vi "composeChipKick.vi"(4 "Game in":refnum<class "Game.lvclass">, 6 "Distance to target":dbl, 8 "error in (no error)":errorcluster, 9 "kick_z":dbl, 10 "kick_x":dbl, 11 "KickToSkill in":refnum<class "KickToSkill.lvclass">) -> (0 "error out":errorcluster, 1 "kick_z out":dbl, 2 "kick_x out":dbl, 3 "KickToSkill out":refnum<class "KickToSkill.lvclass">)   [LabVIEW 2021, in "KickToSkill.lvclass"]
uses:
  KickToSkill.lvclass
  Game_class/Game.lvclass
  Game_class/Game.lvclass/Game.ctl
  Team_class/OffensivePlay.ctl
  Team_class/Team.lvclass/Team.ctl
  Object_class/Object.lvclass/Object.ctl
  <vilib>/Analysis/baseanly.llb/Unit Vector (DBL).vi
  Object_class/Read x.vi
  Team_class/Read OffensivePlay.vi
  Game_class/Read BallRef.vi
  Game_class/Read FieldRef.vi
  Game_class/Read NewParameters.vi
  Game_class/Read OffensiveTeam.vi
  Ball_class/Ball.lvclass
  D:/RoboIme/horie/SSL_AI/Object_class/Object.lvclass
  Ally_class/Ally.lvclass
  D:/RoboIme/horie/SSL_AI/Team_class/Team.lvclass
  Field_class/Field.lvclass
  <vilib>/Analysis/NI_AALBase.lvlib
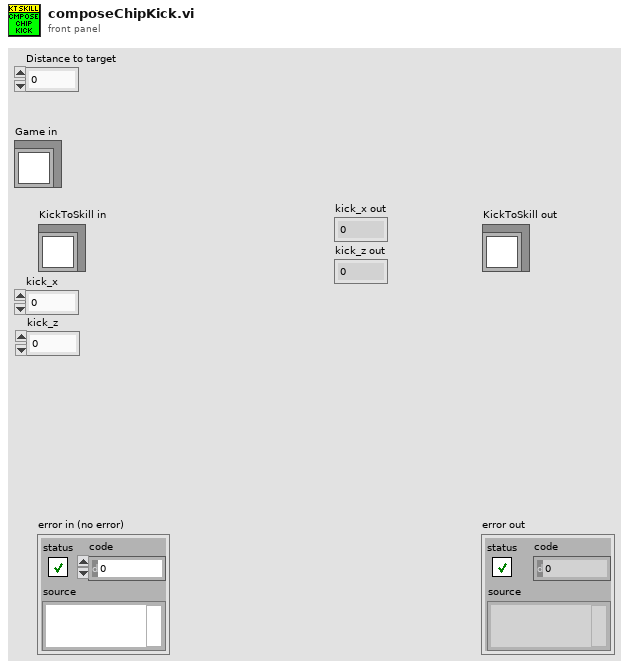
[diagram p1: front panel]
types:
  T1 = typedef "NewParameters.ctl" = cluster{"PenaltyDistance":dbl, "DistanceAttackerToBackBall":dbl, "Division":enum16{"Div B", "Div A"}, "DistanceToAvoidyEnemyRobot":dbl, "BallPlacementDistance":dbl, "DisatanceBehindBallToStealBall":dbl, "MaxDistanceToPositionKickoff":dbl, "BlockEnemyTarget":bool, "MaxStopVAng":dbl, "DistanceMarkerToEnemy":dbl, "IgnoreDribblerContact":bool, "DistanceToBeginEnemyPosession":dbl, "GoToBallWhenEnemyNotMoving":bool, "EnemyDistanceToReduceVelocity":dbl, "TurnOnEnemyDistanceToReduceVelocity":bool, "EnemyDistanceToShootOutBall":dbl, "DefenseKickBall":bool, "MoreKickToGoal? (0-0.3)":dbl, "ChipKickInEnemyField":bool, "ShootOutRobotId":dbl, "FieldLenghtDenominatorInShootOut":dbl, "AdjustPositionInBallPlacement":bool, "PowerGodPass":dbl, "VelocityAbortEnemyPos":dbl, "MaxDistToBeginPass":dbl, "MinDistToBeginPass":dbl, "VelocityInDirects":dbl, "BadDribblerIDs":i32[], "NewKickToDistanceAroundBall":dbl, "PowerAvoidColisionMarker":dbl, "DistanceToAvoidColisionMarker":dbl, "AvoidBallKick":dbl, "DistanceTryKick":dbl, "SuicideKickDIstance":dbl, "FirstKickAtck":bool, "AdjustFirstKickDistance":dbl, "FirstKickDefense":bool, "AvoidAimLessKick":dbl, "DistanceToAvoidyEnemyShootRobot ":dbl, "NumberOfMarkers":dbl, "PotField":bool, "PIDLateral":bool, "MinDistanceFirstKickX":dbl, "MinDistanceFirstKickY":dbl, "FractionOfDistToTouchGround\nAfterChipKick":dbl, "FractionOfKickxWhen\nComposedWithKickz":dbl, "Style":T2, "MoveInTurnState":bool, "DistFromEnemyToConsider\nMoveInTurnState":dbl, "CascadePID":bool, "TurnAroundParameters":cluster{"Radius":dbl, "Multiplier":dbl, "ChordAngle":dbl}, "SafeDriveVel":dbl, "DistanceToGoToBackBall":dbl}
  T2 = typedef "Style.ctl" = enum16{"Insanity", "Offensive", "Defensive"}
  T3 = typedef "OffensivePlay.ctl" = enum16{"5RobotsPassGamePlay", "5PreparePassGame", "5RobotsKeeperGame", "KeeperPassToStriker", "5RobotsNormalGamePlay", "PrepareKeeperPass", "ACBPass", "ABCPass", "PrepareTriplePass", "TableWithStriker", "TableWith2ndStrikerPlay", "PrepareDoublePass", "PrepareRollToPass", "SimplePass", "PreparePass", "PassToStriker", "BallOutOfField", "PassTo2ndStriker", "StopOffensive", "Prepare Penalty Enemy", "EnemyPossessionAtEnemyField", "EnemyPossesionAtOurField", "TestPlay", "PreparePenaltyAlly", "KickPenaltyAlly", "PrepareKickoffAlly", "PrepareKickoffEnemy", "IndirectEnemy", "DirectEnemy", "PreparePassInGame1", "NormalGame", "DirectKick", "Pass", "Halt", "Timeout", "PassPlay", "PenaltyEnemy"}
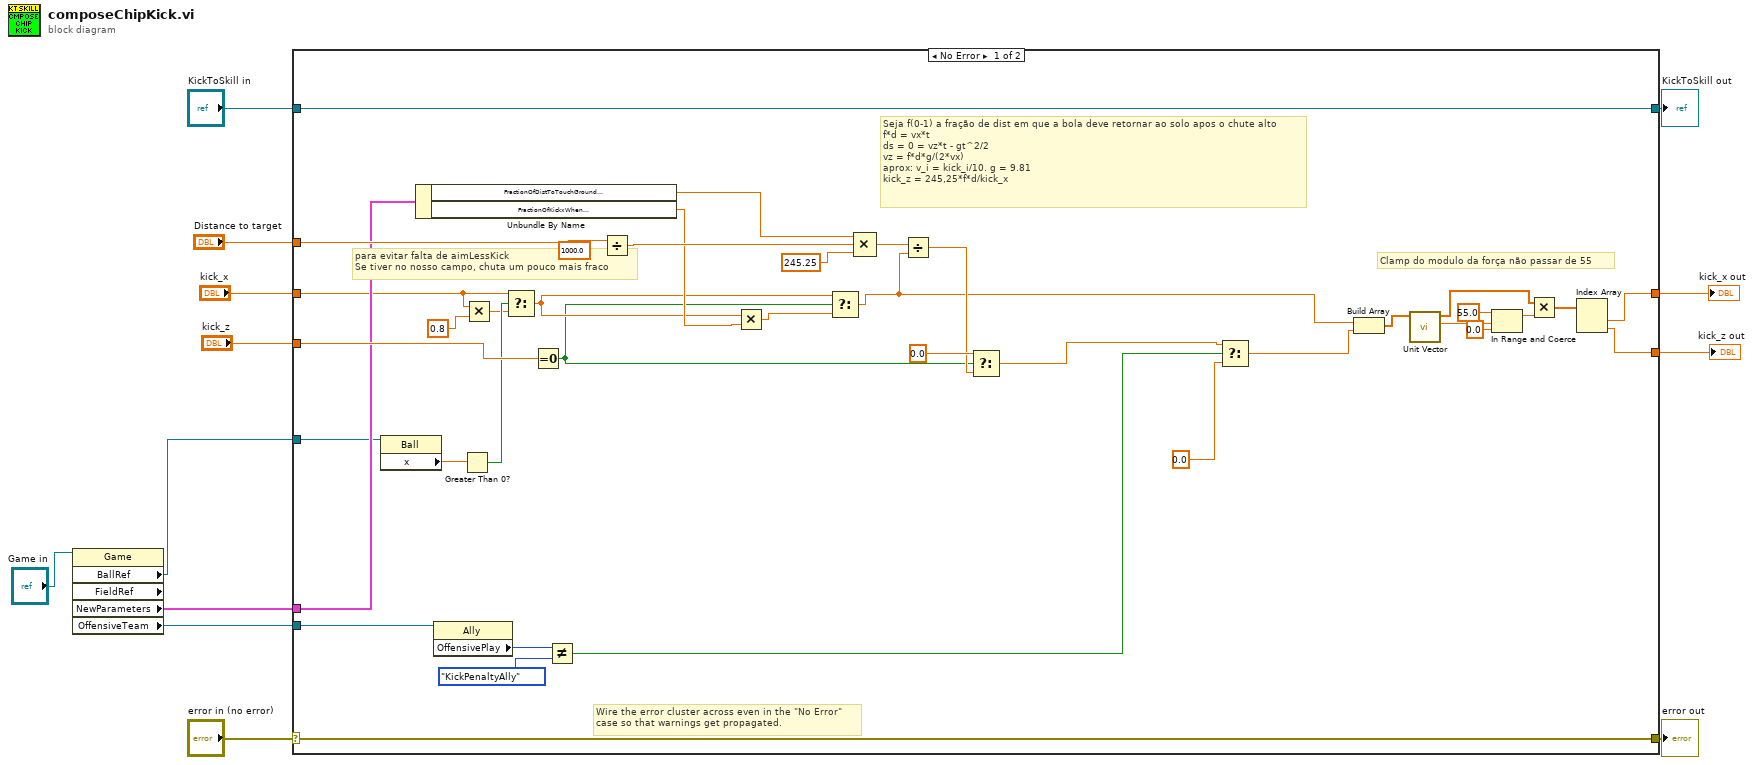
[diagram p0: block diagram]
diagram:
  n1 = property class="Game" props=["BallRef", "FieldRef", "NewParameters", "OffensiveTeam"](reference="Game in") -> ("BallRef"=w1:refnum<class "Ball.lvclass">, "NewParameters"=w4:T1, "OffensiveTeam"=w3:refnum<class "Ally.lvclass">)  [unwired: 1 in, 3 out]
  n2 = case shown="No Error" "error in (no error)" {
    selector: "error in (no error)" -> [w51 w54]
    tunnel: [w51 w54] -> w12
    tunnel: [w52 w53] -> w10
    tunnel: "KickToSkill in" -> [w52 w53]
    tunnel: [w23 _] -> w7
    tunnel: "kick_x" -> [w17 _]
    tunnel: [w22 _] -> w6
    tunnel: "kick_z" -> [w45 _]
    tunnel: w4 -> [w35 _]
    tunnel: w3 -> [w50 _]
    tunnel: "Distance to target" -> [w38 _]
    tunnel: w1 -> [w21 _]
    frame No Error {
      # "para evitar falta de aimLessKick\nSe tiver no nosso campo, chuta um pouco mais fraco"
      # "Clamp do modulo da força não passar de 55"
      # "Seja f(0-1) a fração de dist em que a bola deve retornar ao solo apos o chute alto\nf*d = vx*t \nds = 0 = vz*t - gt^2/2\nvz = f*d*g/(2*vx)\naprox: v_i = kick_i/10. g = 9.81\nkick_z = 245,25*f*d/kick_x"
      # "Wire the error cluster across even in the \"No Error\"\ncase so that warnings get propagated."
      n3 = property class="Ball"(reference=w21) -> ("x"=w20:dbl)  [unwired: 1 in, 2 out]
      n4 = Unbundle By Name(w35) -> ("FractionOfDistToTouchGround\nAfterChipKick"=w34:dbl, "FractionOfKickxWhen\nComposedWithKickz"=w33:dbl)
      n5 = property class="Ally"(reference=w50) -> ("OffensivePlay"=w49:T3)  [unwired: 1 in, 2 out]
      n6 = Greater Than 0?(x=w20) -> (x > 0?=w19:bool)
      n7 = Multiply(x=w17, y=0.8 ("f")) -> (x*y=w18:dbl)
      n8 = Select(t=w17, s=w19, f=w18) -> (s? t:f=w15:dbl)
      n9 = Equal To 0?(x=w45) -> (x = 0?=w14:bool)
      n10 = Not Equal?(x=w49, y=OffensivePlay."KickPenaltyAlly") -> (x != y?=w47:bool)
      n11 = Divide(x=w38, y=1000.0) -> (x/y=w36:dbl)
      n12 = Multiply(x=w15, y=w33) -> (x*y=w44:dbl)
      n13 = Select(t=w15, s=w14, f=w44) -> (s? t:f=w32:dbl)
      n14 = Compound Arithmetic op=MULTIPLY(w34, w36, 245.25) -> (w42:dbl)
      n15 = Divide(x=w42, y=w32) -> (x/y=w40:dbl)
      n16 = Select(t=0.0, s=w14, f=w40) -> (s? t:f=w39:dbl)
      n17 = Select(t=w39, s=w47, f=0.0) -> (s? t:f=w31:dbl)
      n18 = Build Array(w32, w31) -> (w30:dbl[])
      n19 = call-poly <vilib>:"Unit Vector.vi"("Input Vector"=w30) -> ("norm"=w27:dbl, "Unit Vector"=w26:dbl[])  [unwired: 8 in, 1 out]
      n20 = In Range and Coerce(upper limit=55.0, x=w27, lower limit=0.0) -> (coerced(x)=w25:dbl)  [unwired: 1 out]
      n21 = Multiply(x=w26, y=w25) -> (x*y=w24:dbl[])
      n22 = Index Array(array=w24) -> (element #1=w23:dbl, element #2=w22:dbl)  [unwired: 2 in]
    }
    frame Error {
    }
  }
  "error out" <- w12
  "KickToSkill out" <- w10
  "kick_x out" <- w7
  "kick_z out" <- w6
